vi "test3.1-MappingRelationshipByExternalRegistration_API.vi"() -> ()   [LabVIEW 2017, in "testcase-CSMBroadcast.lvclass"]
uses:
  testcase-CSMBroadcast.lvclass
  src/user.lib/_NEVSTOP/Communicable State Machine(CSM)/Communicable State Machine.lvlib
  <vilib>/addons/_JKI Toolkits/VI Tester/TestCase.llb/TestCase.lvclass
  CSM/CSM-Testcase.lvlib
  C:/Program Files (x86)/National Instruments/LabVIEW 2017/vi.lib/addons/_JKI Toolkits/VI Tester/TestCase.llb/TestCase.lvclass
panel:
  out "Loop Count":i32
  out "TestCase out":refnum<class "testcase-CSMBroadcast.lvclass">
  in  "TestCase in":refnum<class "testcase-CSMBroadcast.lvclass">
  out "error out":errorcluster
  in  "error in (no error)":errorcluster
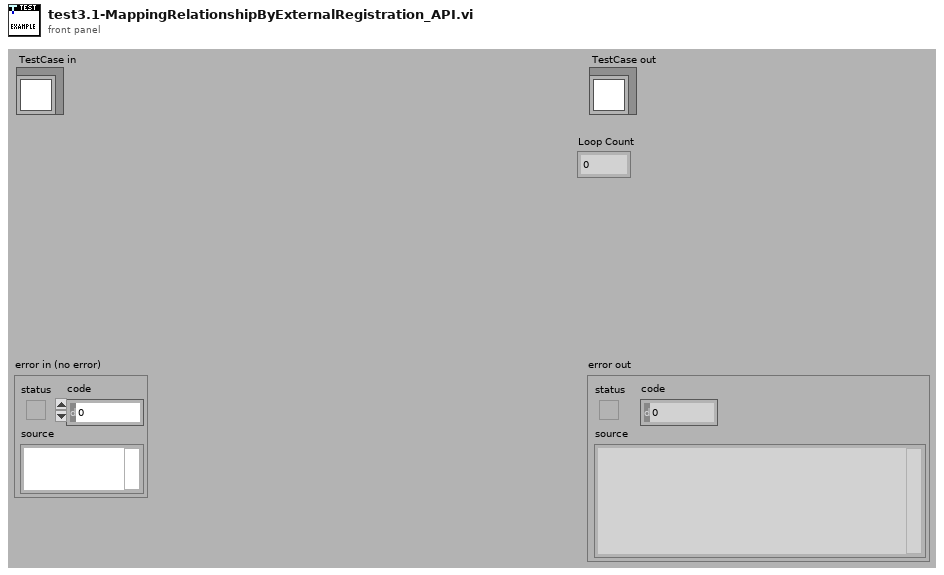
[diagram p1: front panel]
types:
  T1 = cluster{"Status":string, "Source CSM":string, "Target CSM":string, "Target API":string}[]
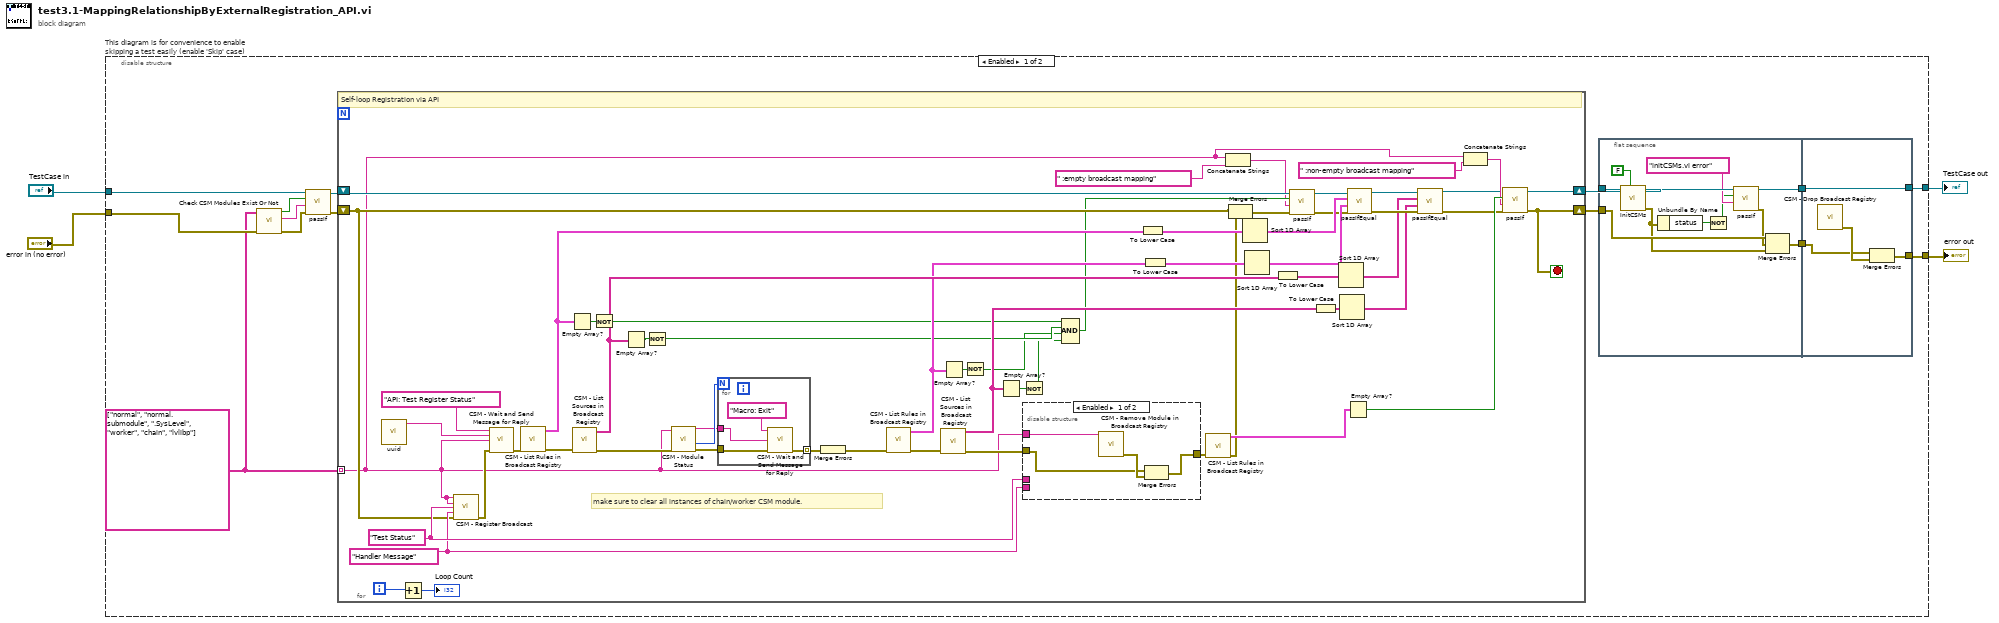
[diagram p0: block diagram]
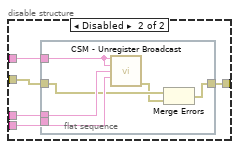
[diagram p2: hidden frame]
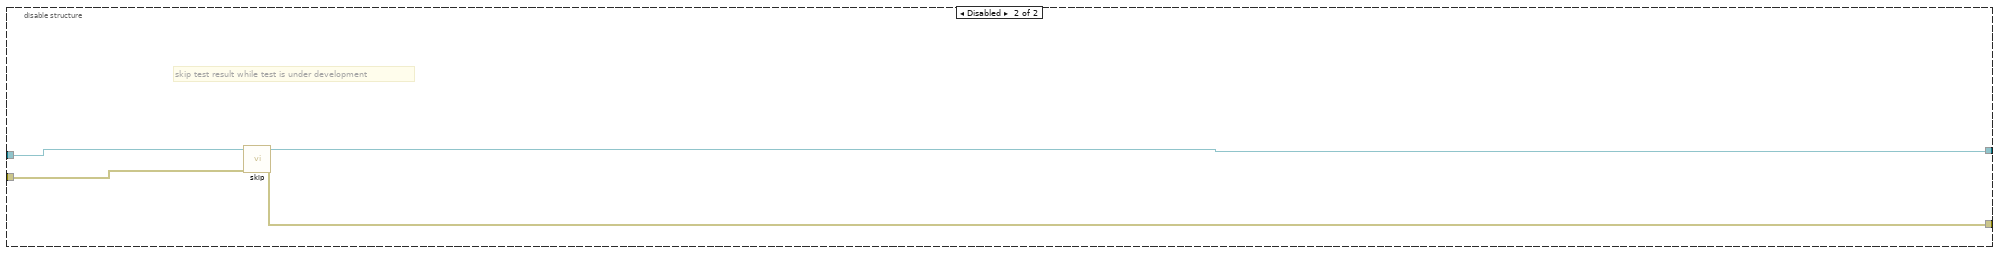
[diagram p3: hidden frame]
diagram:
  n1 = disable-structure "This diagram is for convenience to enable skipping a test easily (enable 'Skip' case)" shown="Enabled" {
    disable-tunnel: "TestCase in" -> [w12 w114]
    disable-tunnel: [w7 w112] -> w1
    disable-tunnel: [w6 w113] -> w3
    disable-tunnel: "error in (no error)" -> [w10 w111]
    frame Enabled {
      w8 = string[] ["normal", "normal.submodule", ".SysLevel", "worker", "chain", "lvlibp"]
      n2 = call "Check CSM Modules Exist Or Not.vi"("error in"=w10, "CSM names in"=w8) -> ("error out"=w13:errorcluster, "Debug string"=w14:string, "All Modules Exist?"=w15:bool)  [unwired: 7 in]
      n3 = call-dynamic "passIf.vi"("error in (no error)"=w13, "message (\"\")"=w14, "pass"=w15, "TestCase in"=w12) -> ("error out"=w9:errorcluster, "TestCase out"=w11:refnum<class "testcase-CSMBroadcast.lvclass">)  [unwired: 6 in]
      n4 = for {
        tunnel: w8 -> [w36] mode=indexing
        shift-right: [w56] -> w17
        shift-left: w11 -> [w40]
        shift-right: [w54] -> w16
        shift-left: w9 -> [w39]
        i -> [w76]
        stop <- w54 stop-if-true
        w59 = "Handler Message" ("Response Message (If \"\", Same as Source Message)")
        w60 = "Test Status" ("Status")
        # "make sure to clear all instances of chain/worker CSM module."
        # "Self-loop Registration via API"
        n5 = call "uuid.vi"() -> ("UUID"=w90:string)  [unwired: 11 in]
        n6 = Increment(x=w76) -> (x+1=→"Loop Count":i32)
        n7 = call "CSM - Register Broadcast.vi"("CSM Name(Empty for Broadcast Event)"=w36, "Source CSM Name (* as Default)"=w36, "Trigger"=w60, "API (If \"\", Same as Trigger)"=w59, "Error In"=w39) -> ("error out"=w61:errorcluster)  [unwired: 9 in, 1 out]
        n8 = call "CSM - Wait and Send Message for Reply.vi"("State"="API: Test Register Status", "Arguments (\"\")"=w90, "Target Module"=w36, "Error In (No Error)"=w61) -> ("error out"=w89:errorcluster)  [unwired: 8 in, 3 out]
        n9 = call "CSM - List Rules in Broadcast Registry.vi"("error in (no error)"=w89) -> ("error out"=w88:errorcluster, "Rule Entries"=w74:T1)  [unwired: 8 in, 1 out]
        n10 = Empty Array?(array=w74) -> (empty?=w73:bool)
        n11 = call "CSM - List Sources in Broadcast Registry.vi"("error in (no error)"=w88) -> ("error out"=w51:errorcluster, "Broadcast Names"=w71:string[])  [unwired: 9 in]
        n12 = Not(x=w73) -> (.not. x?=w66:bool)
        n13 = Empty Array?(array=w71) -> (empty?=w72:bool)
        n14 = Not(x=w72) -> (.not. x?=w65:bool)
        n15 = call "CSM - Module Status.vi"("Error In"=w51, "CSM Name"=w36) -> ("error out"=w50:errorcluster, "#Nodes"=w53:i32, "CSM Name (Dup)"=w52:string)  [unwired: 5 in, 2 out]
        n16 = for {
          N: w53 -> [_]
          tunnel: w52 -> [w94]
          tunnel: w50 -> [w93]
          tunnel: [w92] -> w48 mode=indexing
          n17 = call "CSM - Wait and Send Message for Reply.vi"("State"="Macro: Exit", "Target Module"=w94, "Error In (No Error)"=w93) -> ("error out"=w92:errorcluster)  [unwired: 9 in, 3 out]
        }
        n18 = Merge Errors(w48) -> (w49:errorcluster)
        n19 = call "CSM - List Rules in Broadcast Registry.vi"("error in (no error)"=w49) -> ("error out"=w87:errorcluster, "Rule Entries"=w69:T1)  [unwired: 8 in, 1 out]
        n20 = call "CSM - List Sources in Broadcast Registry.vi"("error in (no error)"=w87) -> ("error out"=w62:errorcluster, "Broadcast Names"=w67:string[])  [unwired: 9 in]
        n21 = Empty Array?(array=w69) -> (empty?=w70:bool)
        n22 = Not(x=w70) -> (.not. x?=w64:bool)
        n23 = Empty Array?(array=w67) -> (empty?=w68:bool)
        n24 = Not(x=w68) -> (.not. x?=w63:bool)
        n25 = disable-structure shown="Enabled" {
          disable-tunnel: w62 -> [w96 w101]
          disable-tunnel: [w97 w100] -> w58
          disable-tunnel: w36 -> [w98 w102]
          disable-tunnel: w60 -> [_ w104]
          disable-tunnel: w59 -> [_ w103]
          frame Enabled {
            n26 = call "CSM - Remove Module in Broadcast Registry.vi"("CSM Name"=w98) -> ("error out"=w99:errorcluster)  [unwired: 13 in, 1 out]
            n27 = Merge Errors(w96, w99) -> (w97:errorcluster)
          }
          frame Disabled {
            n28 = flat-sequence {
              tunnel: w104 -> [w110]
              tunnel: w103 -> [w109]
              tunnel: w102 -> [w108]
              tunnel: w101 -> [w107]
              tunnel: [w105] -> w100
              frame #0 {
                n29 = call "CSM - Unregister Broadcast.vi"("CSM Name(Empty for Broadcast Event)"=w108, "Source CSM Name (* as Default)"=w108, "Trigger"=w110, "API (\"*\" as Default)"=w109) -> ("error out"=w106:errorcluster)  [unwired: 10 in, 1 out]
                n30 = Merge Errors(w107, w106) -> (w105:errorcluster)
              }
            }
          }
        }
        n31 = Compound Arithmetic op=AND(w66, w65, w64, w63) -> (w38:bool)
        n32 = To Lower Case(string=w74) -> (all lower case string=w86:T1)
        n33 = To Lower Case(string=w69) -> (all lower case string=w85:T1)
        n34 = call "CSM - List Rules in Broadcast Registry.vi"("error in (no error)"=w58) -> ("error out"=w46:errorcluster, "Rule Entries"=w57:T1)  [unwired: 8 in, 1 out]
        n35 = Concatenate Strings(w36, " :empty broadcast mapping" ("string")) -> (w37:string)
        n36 = Merge Errors(w39, w46) -> (w43:errorcluster)
        n37 = Sort 1D Array(array=w86) -> (sorted array=w84:T1)
        n38 = Sort 1D Array(array=w85) -> (sorted array=w83:T1)
        n39 = To Lower Case(string=w71) -> (all lower case string=w80:string[])
        n40 = call-dynamic "passIf.vi"("error in (no error)"=w43, "message (\"\")"=w37, "pass"=w38, "TestCase in"=w40) -> ("error out"=w42:errorcluster, "TestCase out"=w41:refnum<class "testcase-CSMBroadcast.lvclass">)  [unwired: 6 in]
        n41 = To Lower Case(string=w67) -> (all lower case string=w79:string[])
        n42 = Sort 1D Array(array=w80) -> (sorted array=w78:string[])
        n43 = Sort 1D Array(array=w79) -> (sorted array=w77:string[])
        n44 = Empty Array?(array=w57) -> (empty?=w55:bool)
        n45 = call-dynamic "passIfEqual.vi"("error in (no error)"=w42, "y"=w83, "x"=w84, "TestCase in"=w41) -> ("error out"=w81:errorcluster, "TestCase out"=w82:refnum<class "testcase-CSMBroadcast.lvclass">)  [unwired: 6 in]
        n46 = call-dynamic "passIfEqual.vi"("error in (no error)"=w81, "y"=w77, "x"=w78, "TestCase in"=w82) -> ("error out"=w34:errorcluster, "TestCase out"=w35:refnum<class "testcase-CSMBroadcast.lvclass">)  [unwired: 6 in]
        n47 = Concatenate Strings(w36, " :non-empty broadcast mapping" ("string")) -> (w44:string)
        n48 = call-dynamic "passIf.vi"("error in (no error)"=w34, "message (\"\")"=w44, "pass"=w55, "TestCase in"=w35) -> ("error out"=w54:errorcluster, "TestCase out"=w56:refnum<class "testcase-CSMBroadcast.lvclass">)  [unwired: 6 in]
      }
      n49 = flat-sequence {
        tunnel: w17 -> [w29]
        tunnel: [w26] -> w18
        tunnel: w16 -> [w23]
        tunnel: [w20] -> w5
        tunnel: w18 -> [w32]
        tunnel: [w32] -> w7
        tunnel: [w31] -> w6
        tunnel: w5 -> [w30]
        frame #0 {
          n50 = call "InitCSMs.vi"("Enable building lvlibp?"=FALSE, "testcase-CSMStatus in"=w29) -> ("error out"=w21:errorcluster, "testcase-CSMStatus out"=w27:refnum<class "testcase-CSMBroadcast.lvclass">)  [unwired: 8 in]
          n51 = Unbundle By Name(w21) -> ("status"=w25:bool)
          n52 = Not(x=w25) -> (.not. x?=w19:bool)
          n53 = call-dynamic "passIf.vi"("message (\"\")"="initCSMs.vi error" ("message (\"\")"), "pass"=w19, "TestCase in"=w27) -> ("error out"=w22:errorcluster, "TestCase out"=w26:refnum<class "testcase-CSMBroadcast.lvclass">)  [unwired: 7 in]
          n54 = Merge Errors(w23, w22, w21) -> (w20:errorcluster)
        }
        frame #1 {
          n55 = call "CSM - Drop Broadcast Registry.vi"() -> ("error out"=w33:errorcluster)  [unwired: 15 in]
          n56 = Merge Errors(w30, w33) -> (w31:errorcluster)
        }
      }
    }
    frame Disabled {
      # "skip test result while test is under development"
      n57 = call <vilib>:"skip.vi"("error in (no error)"=w111, "TestCase in"=w114) -> ("error out"=w113:errorcluster, "TestCase out"=w112:refnum<class "testcase-CSMBroadcast.lvclass">)  [unwired: 8 in]
    }
  }
  "error out" <- w3
  "TestCase out" <- w1
